vi "Terminal_Drive_System_SavetoDB.vi"(8 "error in (no error)":errorcluster caption="错误输入（无错误）", 9 "时间标识":timestamp, 11 "设备信息":T1) -> (3 "error out":errorcluster)   [LabVIEW 2014]
panel:
  in  "停止":bool caption="启动"
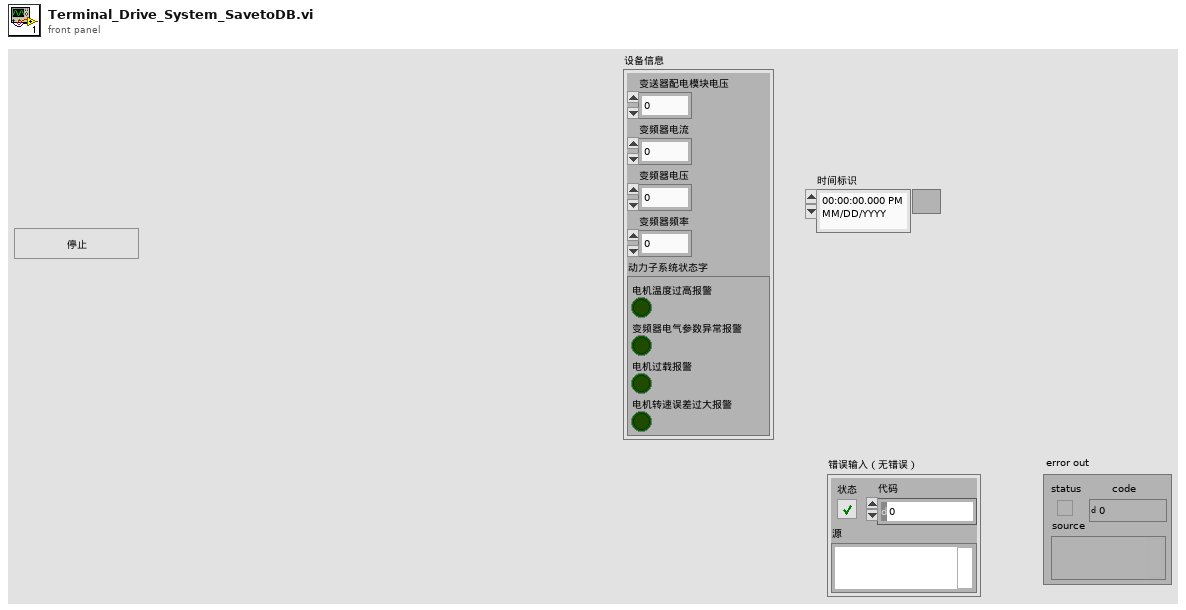
[diagram p1: front panel]
types:
  T1 = cluster{"变送器配电模块电压":u16, "变频器电流":u16, "变频器电压":u16, "变频器频率":u16, "动力子系统状态字":cluster{"电机温度过高报警":bool, "变频器电气参数异常报警":bool, "电机过载报警":bool, "电机转速误差过大报警":bool}}
  T2 = cluster{"变送器配电模块电压":u16, "变频器电流":u16, "变频器电压":u16, "变频器频率":u16}
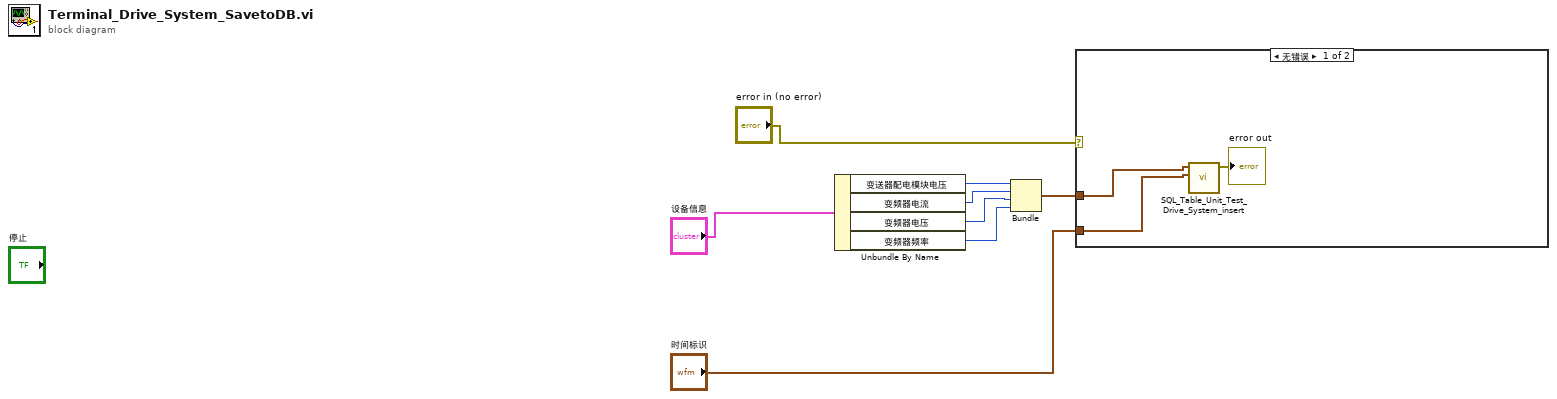
[diagram p0: block diagram]
diagram:
  n1 = Unbundle By Name("设备信息") -> ("变送器配电模块电压"=w8:u16, "变频器电流"=w7:u16, "变频器电压"=w6:u16, "变频器频率"=w5:u16)
  n2 = Bundle("变送器配电模块电压"=w8, "变频器电流"=w7, "变频器电压"=w6, "变频器频率"=w5) -> (w4:T2)  [unwired: 1 in]
  n3 = case shown="无错误" "error in (no error)" {
    tunnel: w4 -> [w11 _]
    tunnel: "时间标识" -> [w10 _]
    frame No Error {
      n4 = call "SQL_Table_Unit_Test_Drive_System_insert.vi"("时间标识"=w10, "动力子系统数据"=w11) -> ("error out"=→"error out":errorcluster)  [unwired: 9 in]
    }
    frame Error {
    }
  }
